vi "PFDE SERVO MOTOR.vi"() -> ()   [LabVIEW 2018]
uses:
  <vilib>/Modbus/master/Create Master Instance (Serial).vi
  <vilib>/Modbus/master/Modbus Master.lvclass
panel:
  in  "转矩调整":u16(slide) scale=0.0..100.0
  out "仪表":u16(knob) scale=0.0..3000.0
  in  "最大转速调整":u16(slide) scale=0.0..3000.0
  in  "启动":bool
  out "内部转矩":u16[](array[numeric])
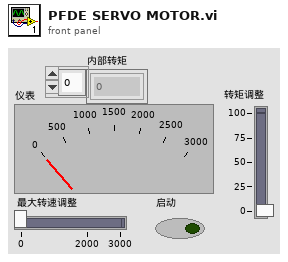
[diagram p1: front panel]
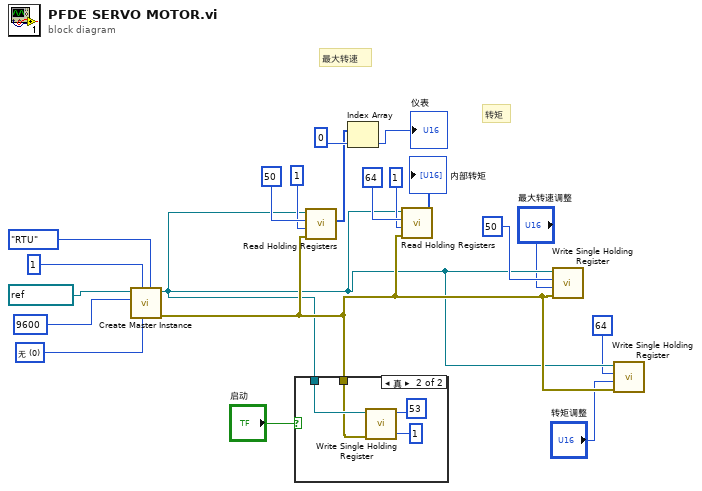
[diagram p0: block diagram]
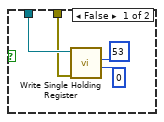
[diagram p2: hidden frame]
diagram:
  w15 = u16 0 items=["无", "奇", "偶"] ("parity (Even)")
  # "转矩"
  # "最大转速"
  n1 = call-poly <vilib>:"Create Master Instance.vi"("serial type"=enum16{"RTU", "ASCII"}."RTU", "parity (Even)"=w15, "unit ID"=u8 1, "baud rate (9600)"=u32 9600, "VISA resource name"=refnum<visa-resource-name> "COM3") -> ("error out"=w6:errorcluster, "serial master instance"=w5:refnum<class "Modbus Master.lvclass">)  [unwired: 5 in]
  n2 = case shown="真" "启动" {
    tunnel: w5 -> [w22 w28]
    tunnel: w6 -> [w21 w26]
    frame False {
      n3 = call-dynamic "Write Single Holding Register.vi"("error in (no error)"=w21, "holding register value"=u16 0, "address"=u16 53, "Modbus master in"=w22) -> ()  [unwired: 6 in, 2 out]
    }
    frame True {
      n4 = call-dynamic "Write Single Holding Register.vi"("error in (no error)"=w26, "holding register value"=u16 1, "address"=u16 53, "Modbus master in"=w28) -> ()  [unwired: 6 in, 2 out]
    }
  }
  n5 = call-dynamic "Read Holding Registers.vi"("error in (no error)"=w6, "number of holding registers"=u16 1, "starting address"=u16 50, "Modbus master in"=w5) -> ("register values"=w1:u16[])  [unwired: 5 in, 2 out]
  n6 = Index Array(array=w1, index=0 ("索引")) -> (element=→"仪表":u16)
  n7 = call-dynamic "Read Holding Registers.vi"("error in (no error)"=w6, "number of holding registers"=u16 1, "starting address"=u16 64, "Modbus master in"=w5) -> ("register values"=→"内部转矩":u16[])  [unwired: 5 in, 2 out]
  n8 = call-dynamic "Write Single Holding Register.vi"("error in (no error)"=w6, "holding register value"="最大转速调整", "address"=u16 50, "Modbus master in"=w5) -> ()  [unwired: 6 in, 2 out]
  n9 = call-dynamic "Write Single Holding Register.vi"("error in (no error)"=w6, "holding register value"="转矩调整", "address"=u16 64 ("holding register value"), "Modbus master in"=w5) -> ()  [unwired: 6 in, 2 out]
